vi "GUI_10TW_HamamatsuDAQ.vi"() -> ()   [LabVIEW 2013]
uses:
  shared programs/GUI_Template/GUI_master/tcp_new_data_event.ctl
  shared programs/GUI_Template/GUI_master/tcp new data cluster.ctl
  <vilib>/Utility/file.llb/Write To Spreadsheet File (DBL).vi
panel:
  in  "Scan#":i32=15585833
  in  "?":enum32{"Raw", "Normalized"}(tab)
  out "Intensity Graph 6":dbl[][](graph)
  out "Intensity Graph 8":dbl[][](graph)
  in  "Last Saved Shot":i32
  in  "trigger::1":bool caption="Trigger"
  in  "stop":bool
  out "Hamamattsu Spectrometer":T1(graph)
  in  "save":bool
  in  "Spectrometer Folder":string="Spectrometer"
  in  "MC Run Directory":path
  in  "shotnum":i32=15585833
  in  "saveFolder":path=path "Z:/10TWdata/Y2011"
  out "Check Save Folder Exists":bool
  in  "MC Save":bool=TRUE
  in  "counts::1":dbl[](array[numeric])
  in  "wavelength::1":dbl[](array[numeric])
  out "tcp data event":T2
  out "error IO 2":errorcluster
  in  "GUIdevice 1":string="10TW HamamatsuDAQ"
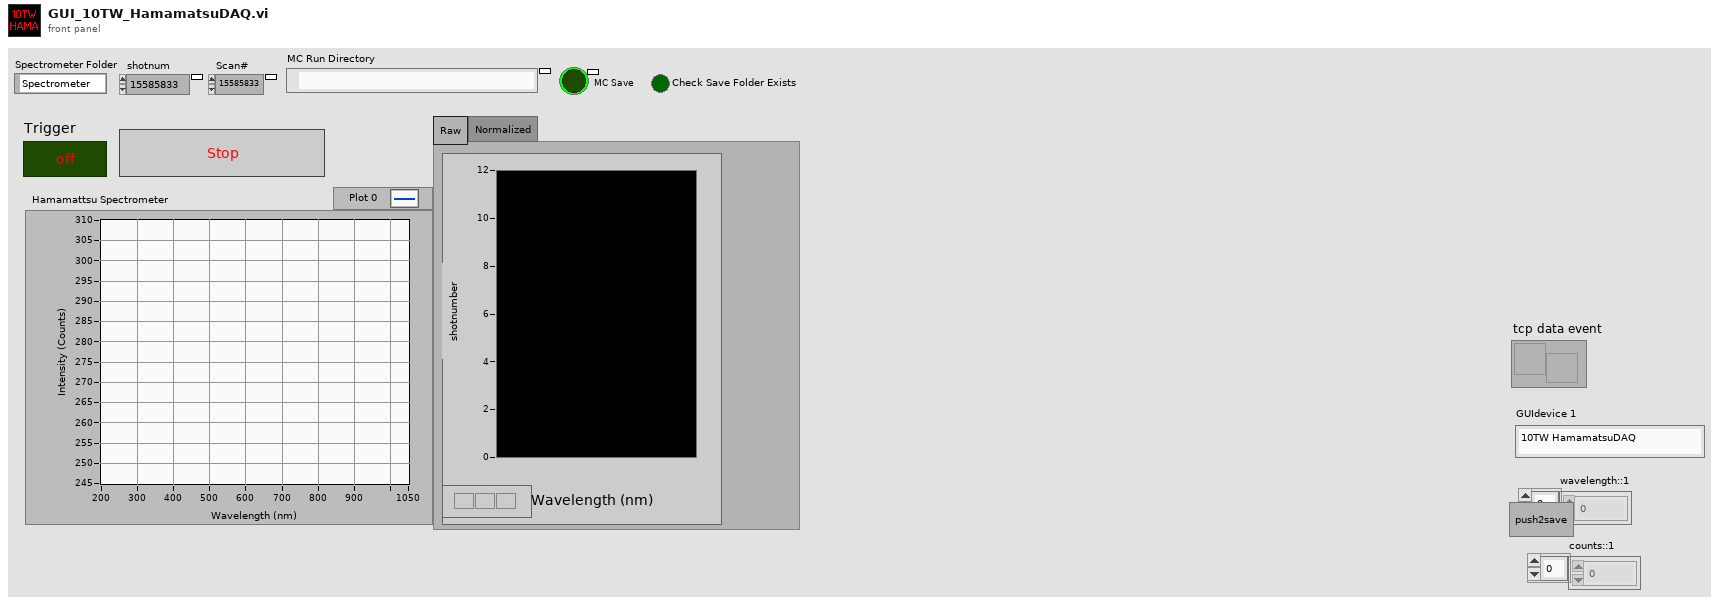
[diagram p1: front panel]
types:
  T1 = cluster{"wavelength::1":dbl[], "counts::1":dbl[]}
  T2 = typedef "tcp_new_data_event.ctl" = refnum<user-event>
  T3 = typedef "tcp new data cluster.ctl" = cluster{"EventEnum":enum16{"new data", "connection status update"}, "Device name":string}
  T4 = typedef "imagedata.ctl" = cluster{"image type":i32, "image depth":i32, "image":u8[], "mask":u8[], "colors":u32[], "Rectangle":cluster{"left":i16, "top":i16, "right":i16, "bottom":i16}}
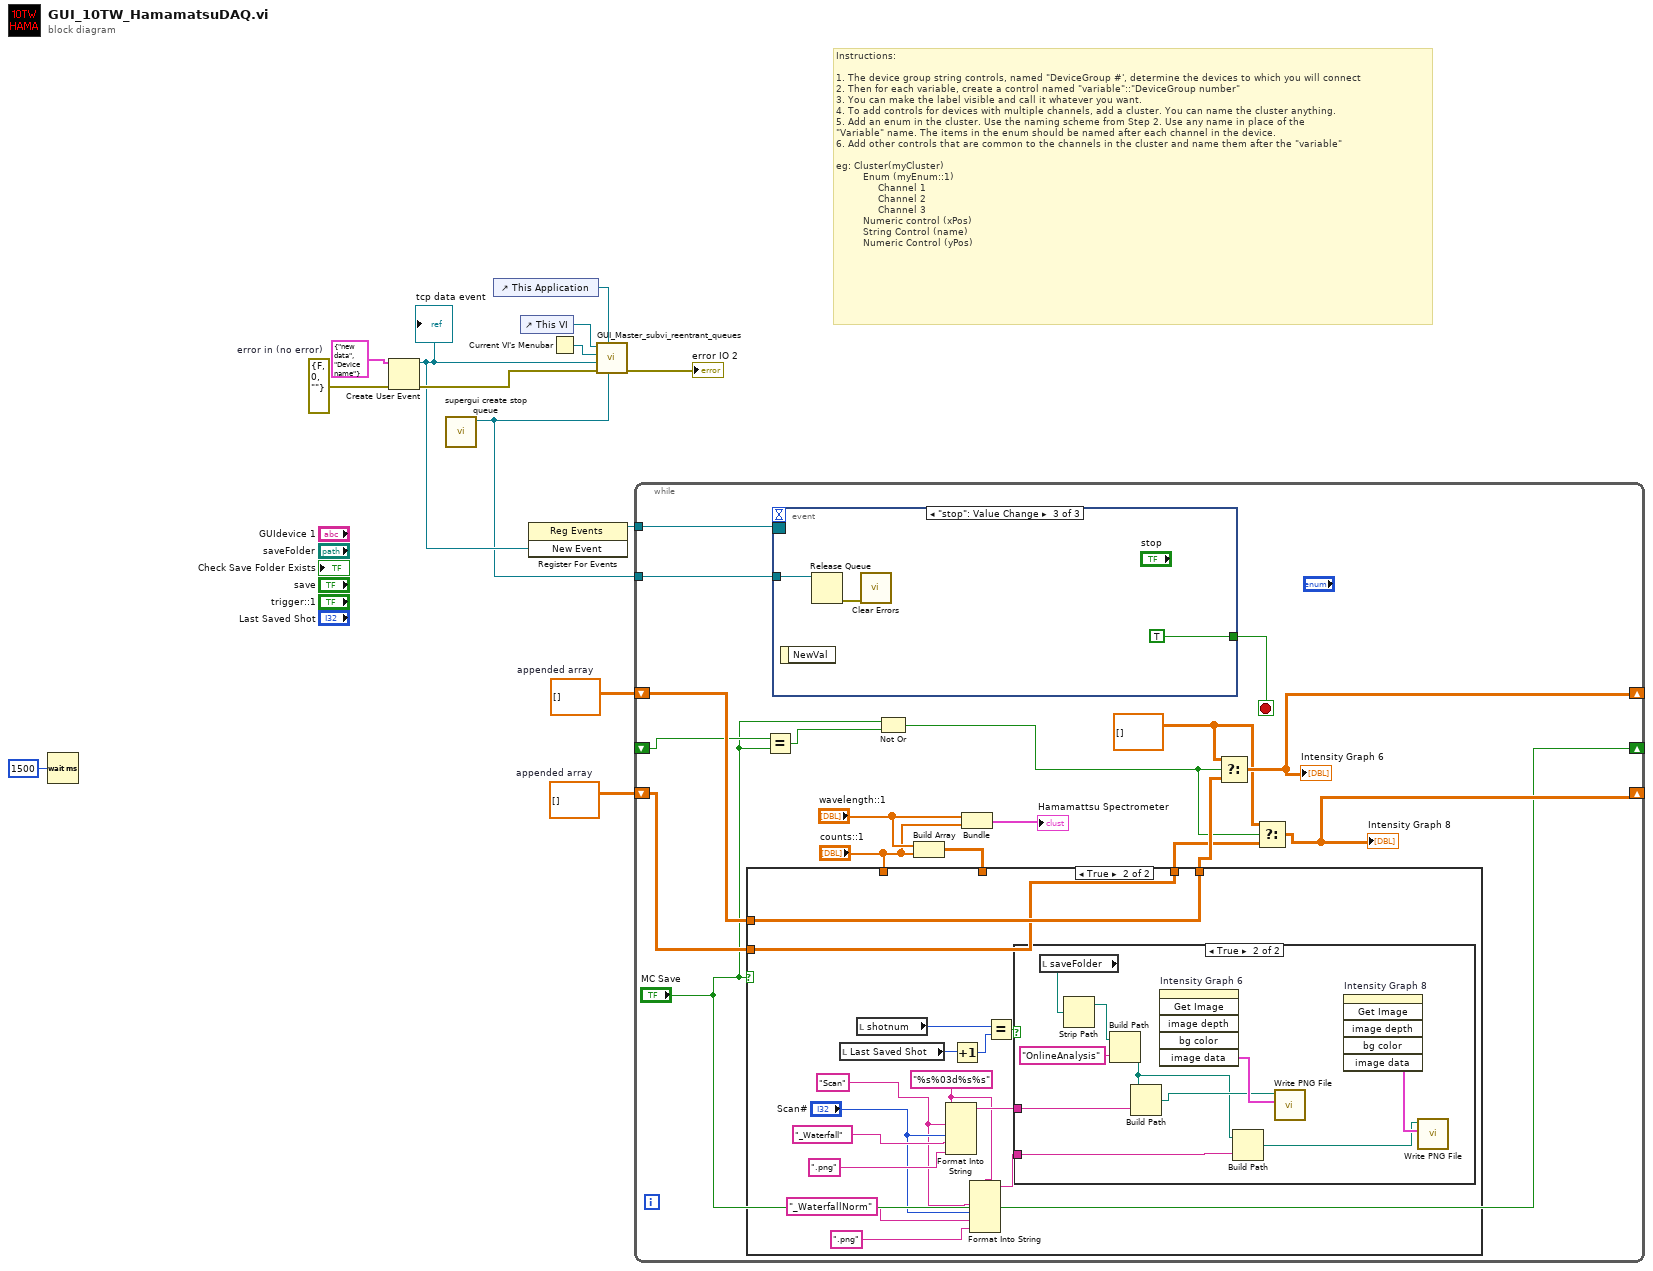
[diagram p0: block diagram]
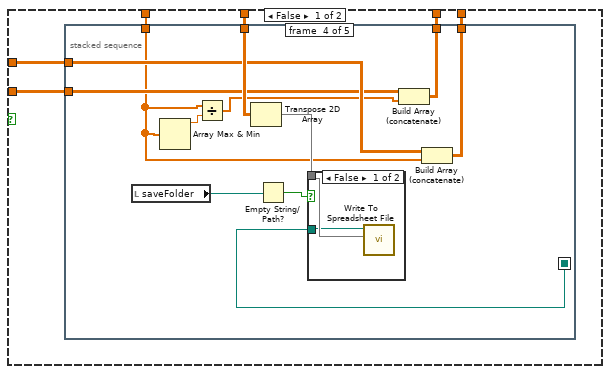
[diagram p2: hidden frame]
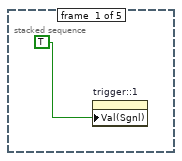
[diagram p3: hidden frame]
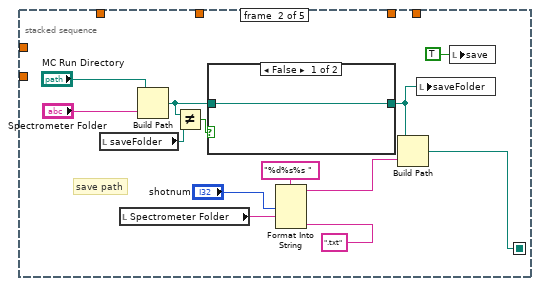
[diagram p4: hidden frame]
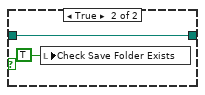
[diagram p5: hidden frame]
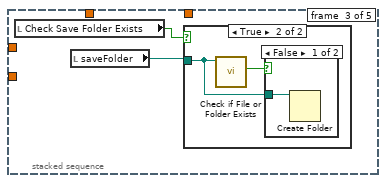
[diagram p6: hidden frame]
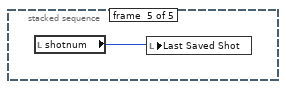
[diagram p10: hidden frame]
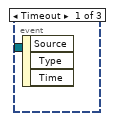
[diagram p12: hidden frame]
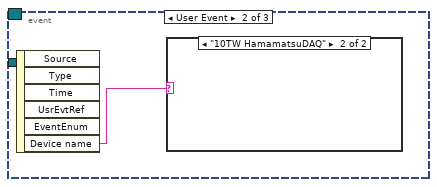
[diagram p13: hidden frame]
diagram:
  w2 = dbl[][] []  # appended array
  w4 = dbl[][] []  # appended array
  w7 = errorcluster {"status"=FALSE, "code"=0, "source"=""}  # error in (no error)
  # "Instructions:\n\n1. The device group string controls, named \"DeviceGroup #', determine the devices to which you will connect\n2. Then for each variable, create a control named \"variable\"::\"DeviceGroup number\"\n3. You can make the label visible and call it whatever you want.\n4. To add controls for devices with multiple channels, add a cluster. You can name the cluster anything.\n5. Add an enum in the cluster. Use the naming scheme from Step 2. Use any name in place of the \n\"Variable\" name. The items in the enum should be named after each channel in the device. \n6. Add other controls that are common to the channels in the cluster and name them after the \"variable\"\n\neg: Cluster(myCluster)\n         Enum (myEnum::1)\n              Channel 1 \n              Channel 2\n              Channel 3\n         Numeric control (xPos)\n         String Control (name)\n         Numeric Control (yPos)"
  n1 = Wait (ms)(milliseconds to wait=u32 1500) -> ()  [unwired: 1 out]
  n2 = Create User Event(user event datatype=T3 {"EventEnum"=enum."new data", "Device name"="Device name"} ("New Event"), error in=w7) -> (user event=w6:refnum<user-event>, error out=w9:errorcluster)
  "tcp data event" <- w6
  n3 = call "supergui create stop queue.vi"() -> ("STOP Queue out"=w1:refnum<queue>)  [unwired: 11 in]
  n4 = control-ref of="This Application"() -> (w8:refnum<vi>)
  n5 = control-ref of="This VI"() -> (w12:refnum<vi>)
  n6 = register-events(w6) -> (reference out=w5:refnum<event-registration>)  [unwired: 2 in, 1 out]
  n7 = Current VI's Menubar() -> (w11:refnum<k9>)
  n8 = call "GUI_Master_subvi_reentrant_queues.vi"("STOP Queue in"=w1, "This Application"=w8, "error in (no error)"=w9, "tcp data event"=w6, "Caller menu reference"=w11, "Caller VI ref"=w12) -> ("error out"=→"error IO 2":errorcluster)  [unwired: 5 in]
  n9 = while {
    tunnel: w5 -> [w31]
    shift-right: [w21] -> _
    shift-left: w4 -> [w26]
    shift-right: ["MC Save"] -> _
    shift-left: _ -> [w24]
    shift-right: [w16] -> _
    shift-left: w2 -> [w20]
    tunnel: w1 -> [w14]
    stop <- w30 stop-if-true
    w17 = dbl[][] [] ("appended array")
    n10 = Equal?(x=w24, y="MC Save") -> (x = y?=w23:bool)
    n11 = event shown="[2] \"stop\": Value Change" {
      selector: w31 -> [_ _ _]
      dyn-events: _ -> [_ _ _]
      timeout: _ -> [_ _ _]
      tunnel: [_ _ TRUE] -> w30
      tunnel: w14 -> [_ _ w102]
      event Timeout {
        n12 = event-data() -> ()  [unwired: 1 in, 3 out]
      }
      event User Event {
        n13 = event-data() -> ("Device name"=w100:string)  [unwired: 1 in, 5 out]
        n14 = case shown="\"10TW HamamatsuDAQ\"" w100 {
          frame "False", Default {
          }
          frame "10TW HamamatsuDAQ" {
          }
        }
      }
      event "stop": Value Change {
        n15 = event-data() -> ()  [unwired: 1 in, 1 out]
        n16 = Release Queue(queue=w102) -> (error out=w101:errorcluster)  [unwired: 2 in, 2 out]
        n17 = call <vilib>:"Clear Errors.vi"("error in (no error)"=w101) -> ()  [unwired: 6 in, 1 out]
      }
    }
    n18 = Not Or(1:w23, 2:"MC Save") -> (0:w18:bool)
    n19 = Build Array("wavelength::1", "counts::1") -> (w27:dbl[][])
    n20 = case shown="True" "MC Save" {
      tunnel: w27 -> [w37 _]
      tunnel: w26 -> [w36 w85]
      tunnel: [w35 w85] -> w22
      tunnel: "counts::1" -> [w34 _]
      tunnel: w20 -> [w33 w83]
      tunnel: [w32 w83] -> w19
      frame False {
        n21 = stacked-sequence {
          seq-local: [_ w41 _ _ _] -> [_ _ _ w67 _]
          tunnel: w37 -> [_ _ _ w70 _]
          tunnel: w36 -> [_ _ _ w68 _]
          tunnel: [_ _ _ w69 _] -> w35
          tunnel: w34 -> [_ _ _ w61 _]
          tunnel: w33 -> [_ _ _ w64 _]
          tunnel: [_ _ _ w63 _] -> w32
          frame #0 {
            n22 = property on="trigger::1" class="Bool (strict)"("Val(Sgnl)"=TRUE ("trigger::1")) -> ()  [unwired: 2 in, 2 out]
          }
          frame #1 {
            # "save path"
            n23 = local read "saveFolder"() -> (w49:path)
            n24 = local read "Spectrometer Folder"() -> (w44:string)
            n25 = Build Path(base path="MC Run Directory", name or relative path="Spectrometer Folder") -> (appended path=w51:path)
            n26 = Not Equal?(x=w51, y=w49) -> (x != y?=w50:bool)
            n27 = case shown="False" w50 {
              tunnel: w51 -> [w52 w54]
              tunnel: [w52 w54] -> w39
              frame False {
              }
              frame True {
                n28 = local write "Check Save Folder Exists"(TRUE ("Check Save Folder Exists")) -> ()
              }
            }
            n29 = Format Into String(format string="%d%s%s ", "shotnum", w44, ".txt" ("input 2")) -> (resulting string=w45:string)  [unwired: 2 in, 1 out]
            n30 = Build Path(base path=w39, name or relative path=w45) -> (appended path=w41:path)
            n31 = local write "saveFolder"(w39) -> ()
            n32 = local write "save"(TRUE ("save")) -> ()
          }
          frame #2 {
            n33 = local read "Check Save Folder Exists"() -> (w56:bool)
            n34 = local read "saveFolder"() -> (w55:path)
            n35 = case shown="True" w56 {
              tunnel: w55 -> [_ w57]
              frame False {
              }
              frame True {
                n36 = call <vilib>:"Check if File or Folder Exists.vi"("path"=w57) -> ("file or folder exists?"=w58:bool)  [unwired: 8 in, 2 out]
                n37 = case shown="False" w58 {
                  tunnel: w57 -> [w59 _]
                  frame False {
                    n38 = Create Folder(path (use dialog)=w59) -> ()  [unwired: 2 in, 3 out]
                  }
                  frame True {
                  }
                }
              }
            }
          }
          frame #3 {
            n39 = local read "saveFolder"() -> (w65:path)
            n40 = Array Max & Min(array=w61) -> (max value=w62:dbl)  [unwired: 3 out]
            n41 = Divide(x=w61, y=w62) -> (x/y=w60:dbl[])
            n42 = Transpose 2D Array(2D array=w70) -> (transposed array=w71:dbl[][])
            n43 = Empty String/Path?(string/path=w65) -> (empty?=w66:bool)
            n44 = case shown="False" w66 {
              tunnel: w71 -> [w73 _]
              tunnel: w67 -> [w72 _]
              frame False {
                n45 = call-poly <vilib>:"Write To Spreadsheet File.vi"("2D data"=w73, "file path (dialog if empty)"=w72) -> ()  [unwired: 6 in, 1 out]
              }
              frame True {
              }
            }
            n46 = Build Array (concatenate)(w64, w60) -> (w63:dbl[][])
            n47 = Build Array (concatenate)(w68, w61) -> (w69:dbl[][])
          }
          frame #4 {
            n48 = local read "shotnum"() -> (w74:i32)
            n49 = local write "Last Saved Shot"(w74) -> ()
          }
        }
      }
      frame True {
        w75 = "Scan" ("input 2")
        w80 = "%s%03d%s%s" ("format string")
        n50 = local read "Last Saved Shot"() -> (w89:i32)
        n51 = local read "shotnum"() -> (w87:i32)
        n52 = Format Into String(format string=w80, w75, "Scan#", "_Waterfall" ("input 2"), ".png" ("input 2")) -> (resulting string=w84:string)  [unwired: 2 in, 1 out]
        n53 = Increment(x=w89) -> (x+1=w88:i32)
        n54 = Format Into String(format string=w80, w75, "Scan#", "_WaterfallNorm" ("input 2"), ".png" ("input 2")) -> (resulting string=w79:string)  [unwired: 2 in, 1 out]
        n55 = Equal?(x=w87, y=w88) -> (x = y?=w86:bool)
        n56 = case shown="True" w86 {
          tunnel: w84 -> [_ w98]
          tunnel: w79 -> [_ w90]
          frame False {
          }
          frame True {
            n57 = local read "saveFolder"() -> (w94:path)
            n58 = Strip Path(path=w94) -> (stripped path=w93:path)  [unwired: 1 out]
            n59 = Build Path(base path=w93, name or relative path="OnlineAnalysis") -> (appended path=w91:path)
            n60 = Build Path(base path=w91, name or relative path=w98) -> (appended path=w97:path)
            n61 = invoke on="Intensity Graph 6" class="IntGraph (strict)" method="Get Image"() -> ("image data"=w99:T4)  [unwired: 6 in, 5 out]
            n62 = Build Path(base path=w91, name or relative path=w90) -> (appended path=w95:path)
            n63 = call <vilib>:"Write PNG File.vi"("image data"=w99, "path to PNG file"=w97) -> ()  [unwired: 8 in, 2 out]
            n64 = invoke on="Intensity Graph 8" class="IntGraph (strict)" method="Get Image"() -> ("image data"=w96:T4)  [unwired: 6 in, 5 out]
            n65 = call <vilib>:"Write PNG File.vi"("image data"=w96, "path to PNG file"=w95) -> ()  [unwired: 8 in, 2 out]
          }
        }
      }
    }
    n66 = Bundle("wavelength::1"="wavelength::1", "counts::1"="counts::1") -> (→"Hamamattsu Spectrometer":T1)  [unwired: 1 in]
    n67 = Select(t=w17, s=w18, f=w22) -> (s? t:f=w21:dbl[][])
    "Intensity Graph 6" <- w21
    n68 = Select(t=w17, s=w18, f=w19) -> (s? t:f=w16:dbl[][])
    "Intensity Graph 8" <- w16
  }
